vi "Panel.vi"(8 "error in (no error)":errorcluster, 9 "Parent Panel Name":string caption="Parent Panel Name (None)", 11 "Panel in":refnum<class "Panel.lvclass">) -> (0 "error out":errorcluster, 3 "Panel out":refnum<class "Panel.lvclass">)   [LabVIEW 2023, in "Panel Actor.lvlib" / "Panel.lvlib" / "Panel.lvclass"]
doc: "Creates a new Panel.\n\nIf <b>Autoshow?</b> is TRUE, then the panel will be shown immediately after initialization. If it is FALSE, the the Show method must be called manually.\n----\nCopyright: MGI 2016\nAuthor: Derek Trepanier"
uses:
  Panel.lvclass
  Panel.lvclass/Panel.ctl
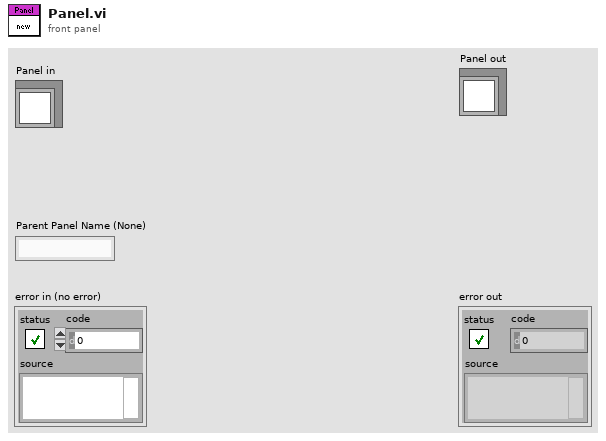
[diagram p1: front panel]
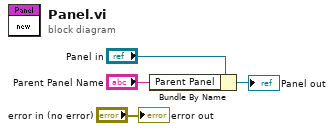
[diagram p0: block diagram]
diagram:
  n1 = Bundle By Name(cluster="Panel in", "Parent Panel"="Parent Panel Name") -> (→"Panel out":refnum<class "Panel.lvclass">)
  "error out" <- "error in (no error)"
